vi "LibraryPathFGV.vi"(1 "Action":enum16{"Read", "Write"}(ring), 5 "Path In":path, 11 "error in (no error)":errorcluster) -> (6 "Path Out":path, 15 "error out":errorcluster)   [LabVIEW 2020, in "fgt_SDK.lvlib"]
uses:
  fgt_SDK.lvlib
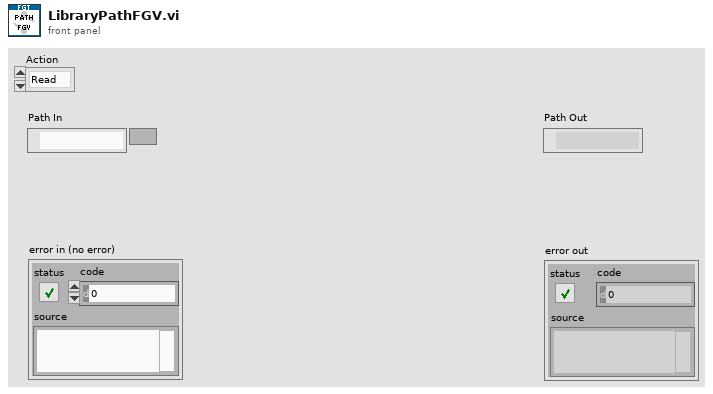
[diagram p1: front panel]
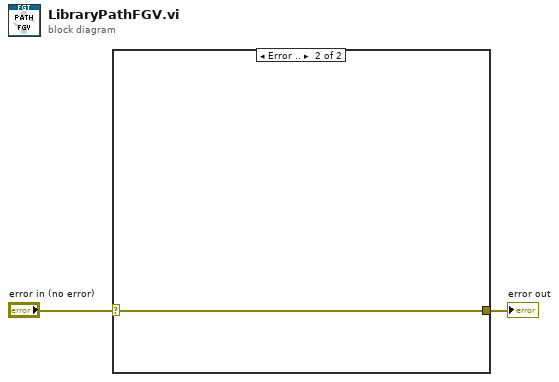
[diagram p0: block diagram]
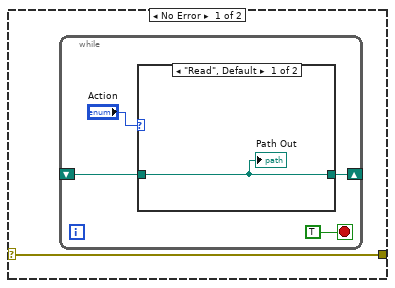
[diagram p2: hidden frame]
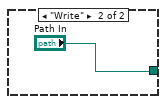
[diagram p3: hidden frame]
diagram:
  n1 = case shown="Error .." "error in (no error)" {
    selector: "error in (no error)" -> [w3 w10]
    tunnel: [w3 w10] -> w1
    frame No Error {
      n2 = while {
        shift-right: [w5] -> _
        shift-left: _ -> [w4]
        stop <- TRUE stop-if-true
        n3 = case shown="\"Read\", Default" "Action" {
          tunnel: [w8 "Path In"] -> w5
          tunnel: w4 -> [w8 _]
          frame "Read", Default {
            "Path Out" <- w8
          }
          frame "Write" {
          }
        }
      }
    }
    frame Error {
    }
  }
  "error out" <- w1
